vi "CRYPEAQ FindPeak.vi"(10 "N":i32, 11 "c2":dbl[](array[numeric])) -> (2 "Index":i32, 3 "cmax(EHS)":dbl)   [LabVIEW 2013]
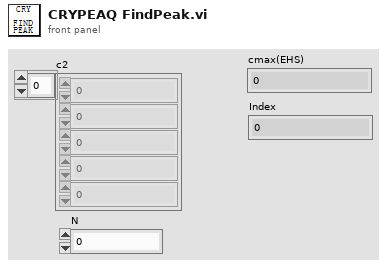
[diagram p1: front panel]
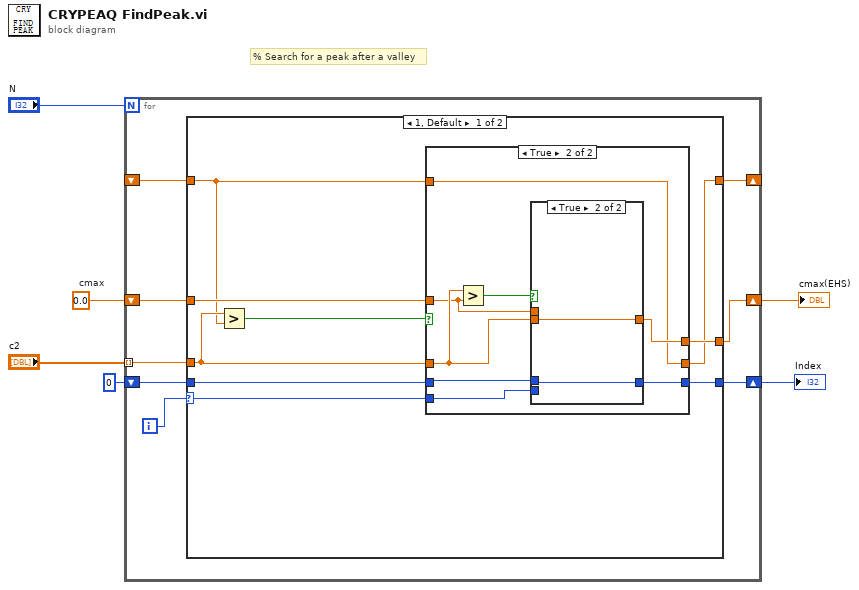
[diagram p0: block diagram]
diagram:
  w6 = 0.0  # cmax
  # "% Search for a peak after a valley"
  n1 = for {
    N: "N" -> [_]
    tunnel: "c2" -> [w13] mode=indexing
    shift-right: [w12] -> _
    shift-left: _ -> [w11]
    shift-right: [w9] -> w5
    shift-left: w6 -> [w10]
    shift-right: [w8] -> w3
    shift-left: 0 -> [w7]
    i -> [w14]
    n2 = case shown="1, Default" w14 {
      selector: w14 -> [w16 w39]
      tunnel: [w18 w41] -> w12
      tunnel: w13 -> [w23 w41]
      tunnel: w11 -> [w17 _]
      tunnel: w10 -> [w22 w40]
      tunnel: [w21 w40] -> w9
      tunnel: [w20 w39] -> w8
      tunnel: w7 -> [w19 _]
      frame 1, Default {
        n3 = Greater?(x=w23, y=w17) -> (0:w15:bool)
        n4 = case shown="True" w15 {
          tunnel: w23 -> [w24 w33]
          tunnel: w22 -> [w26 w31]
          tunnel: [w26 w32] -> w21
          tunnel: [w25 w29] -> w20
          tunnel: w19 -> [w25 w28]
          tunnel: w16 -> [_ w30]
          tunnel: [w24 w27] -> w18
          tunnel: w17 -> [_ w27]
          frame False {
          }
          frame True {
            n5 = Greater?(x=w33, y=w31) -> (0:w34:bool)
            n6 = case shown="True" w34 {
              tunnel: w33 -> [_ w37]
              tunnel: [w36 w37] -> w32
              tunnel: w31 -> [w36 _]
              tunnel: w30 -> [_ w38]
              tunnel: [w35 w38] -> w29
              tunnel: w28 -> [w35 _]
              frame False {
              }
              frame True {
              }
            }
          }
        }
      }
      frame 0 {
      }
    }
  }
  "cmax(EHS)" <- w5
  "Index" <- w3
